vi "Initialize.vi"(8 "error in (no error)":errorcluster) -> (0 "error out":errorcluster, 3 "TCP Reader out":refnum<class "TCP Reader.lvclass">)   [LabVIEW 2018, in "TCP Classes.lvlib" / "TCP Reader.lvclass"]
uses:
  TCP Reader.lvclass
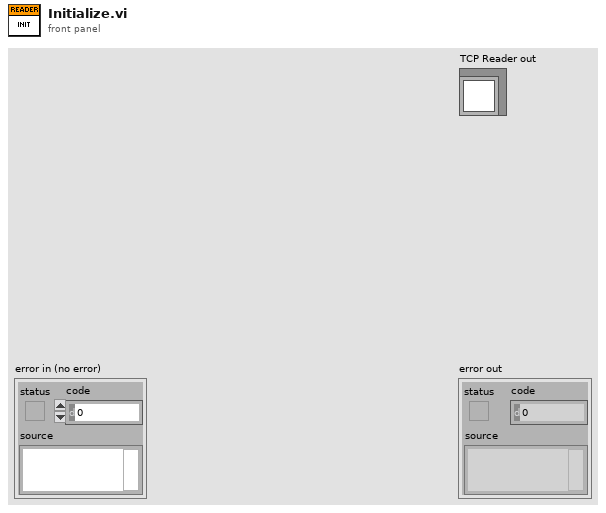
[diagram p1: front panel]
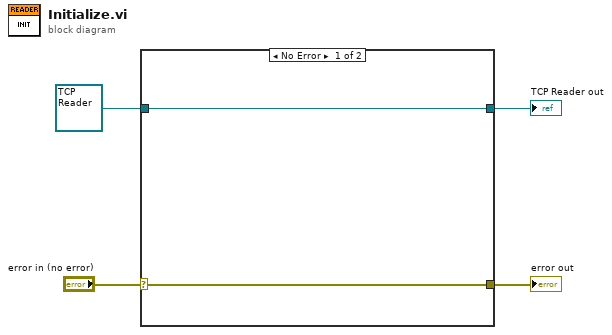
[diagram p0: block diagram]
diagram:
  n1 = case shown="No Error" "error in (no error)" {
    selector: "error in (no error)" -> [w5 w8]
    tunnel: [w5 w8] -> w3
    tunnel: [w6 w7] -> w1
    tunnel: refnum<class "TCP Reader.lvclass"> refnum ("TCP Reader in") -> [w6 w7]
    frame No Error {
    }
    frame Error {
    }
  }
  "error out" <- w3
  "TCP Reader out" <- w1
